vi "Receive.vi"(8 "error in (no error)":errorcluster, 10 "timeout in ms (-1)":i32=-1, 11 "result_from_call in":refnum<class "result_from_call.lvclass">) -> (0 "error out":errorcluster, 2 "timeout":bool, 3 "result_from_call out":refnum<class "result_from_call.lvclass">)   [LabVIEW 2015, in "result_from_call.lvclass"]
uses:
  result_from_call.lvclass
  result_from_call.lvclass/result_from_call.ctl
  result.lvclass
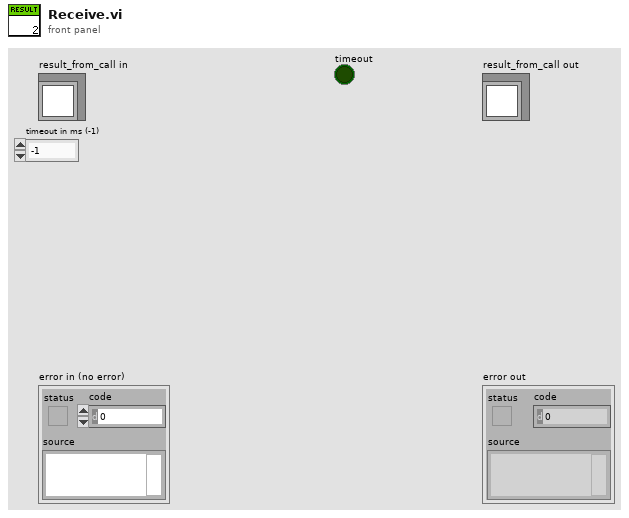
[diagram p1: front panel]
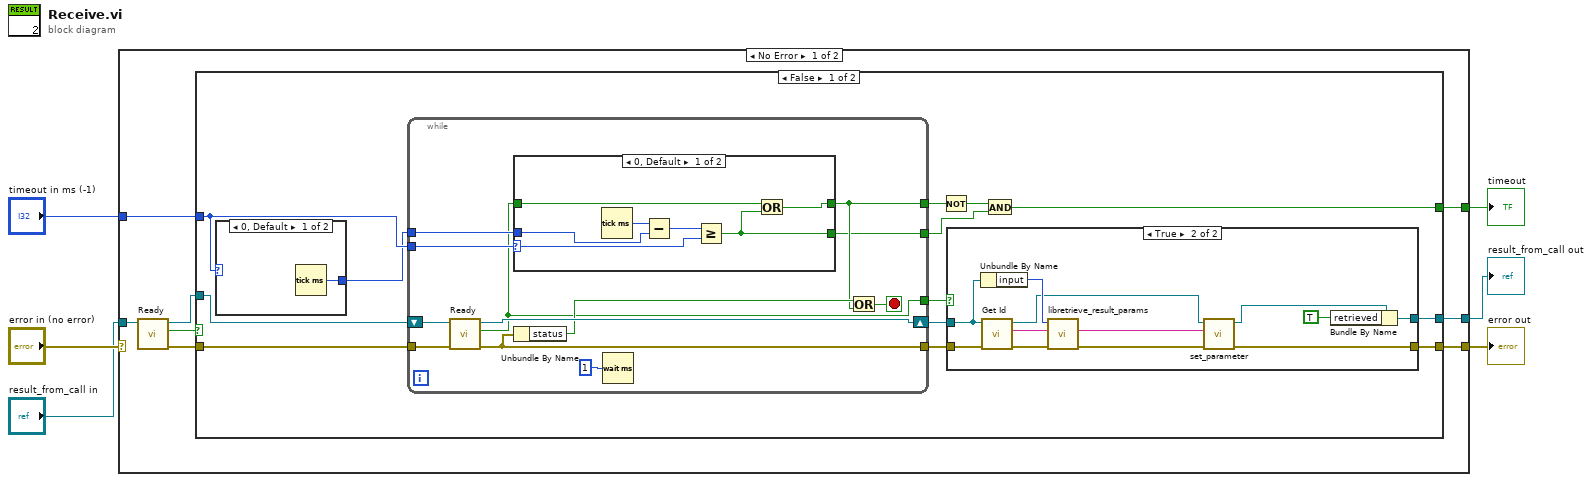
[diagram p0: block diagram]
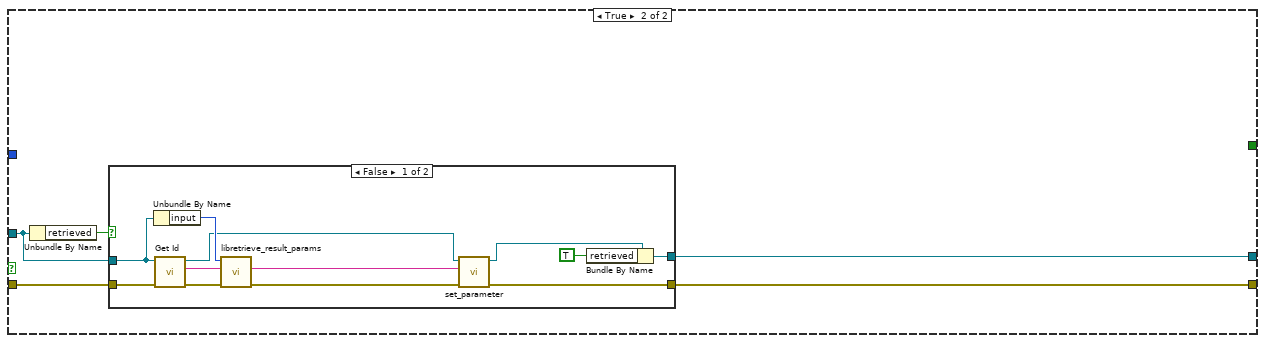
[diagram p5: hidden frame]
diagram:
  n1 = case shown="No Error" "error in (no error)" {
    selector: "error in (no error)" -> [_ w83]
    tunnel: [w13 w83] -> w5
    tunnel: [w12 w82] -> w3
    tunnel: "result_from_call in" -> [w10 w82]
    tunnel: "timeout in ms (-1)" -> [w14 _]
    tunnel: [w11 _] -> w1
    frame No Error {
      n2 = call "Ready.vi"("result_from_call in"=w10) -> ("result_from_call out"=w9:refnum<class "result_from_call.lvclass">, "ready"=w7:bool, "error out"=w8:errorcluster)  [unwired: 7 in]
      n3 = case shown="False" w7 {
        tunnel: w14 -> [w27 _]
        tunnel: [w15 w63] -> w13
        tunnel: [w16 w64] -> w12
        tunnel: [w22 _] -> w11
        tunnel: w9 -> [w21 w65]
        tunnel: w8 -> [w20 w66]
        frame False {
          n4 = case shown="0, Default" w27 {
            tunnel: [w42 _] -> w26
            frame 0, Default {
              n5 = Tick Count (ms)() -> (millisecond timer value=w42:u32)
            }
            frame -1 {
            }
          }
          n6 = while {
            shift-right: [w50] -> w18
            shift-left: w21 -> [w51]
            tunnel: w27 -> [w53]
            tunnel: w26 -> [w52]
            tunnel: [w47] -> w17
            tunnel: [w46] -> w25
            tunnel: [w45] -> w24
            tunnel: w20 -> [w44]
            tunnel: [w43] -> w19
            stop <- w48 stop-if-true
            n7 = call "Ready.vi"("result_from_call in"=w51, "error in (no error)"=w44) -> ("result_from_call out"=w50:refnum<class "result_from_call.lvclass">, "ready"=w43:bool, "error out"=w47:errorcluster)  [unwired: 6 in]
            n8 = case shown="0, Default" w53 {
              selector: w53 -> [w58 _]
              tunnel: w52 -> [w61 _]
              tunnel: w43 -> [w57 w62]
              tunnel: [w56 w62] -> w46
              tunnel: [w55 _] -> w45
              frame 0, Default {
                n9 = Tick Count (ms)() -> (millisecond timer value=w60:u32)
                n10 = Subtract(x=w60, y=w61) -> (x-y=w59:u32)
                n11 = Greater Or Equal?(x=w59, y=w58) -> (x >= y?=w55:bool)
                n12 = Or(x=w57, y=w55) -> (x .or. y?=w56:bool)
              }
              frame -1 {
              }
            }
            n13 = Unbundle By Name(w47) -> ("status"=w49:bool)
            n14 = Wait (ms)(milliseconds to wait=u32 1) -> ()  [unwired: 1 out]
            n15 = Or(x=w49, y=w46) -> (x .or. y?=w48:bool)
          }
          n16 = Not(x=w25) -> (.not. x?=w23:bool)
          n17 = case shown="True" w19 {
            tunnel: w18 -> [w29 w34]
            tunnel: w17 -> [w28 w33]
            tunnel: [w29 w37] -> w16
            tunnel: [w28 w39] -> w15
            frame False {
            }
            frame True {
              n18 = Unbundle By Name(w34) -> ("input"=w35:i32)
              n19 = call "Get Id.vi"("error in (no error)"=w33, "result in"=w34) -> ("error out"=w32:errorcluster, "id"=w31:string, "result out"=w30:refnum<class "result_from_call.lvclass">)  [unwired: 7 in]
              n20 = call "libretrieve_result_params.vi"("error in (no error)"=w32, "id"=w31, "input"=w35) -> ("error out"=w40:errorcluster, "params"=w41:string)  [unwired: 7 in]
              n21 = call "set_parameter.vi"("error in (no error)"=w40, "parameter"=w41, "result in"=w30) -> ("error out"=w39:errorcluster, "result out"=w38:refnum<class "result_from_call.lvclass">)  [unwired: 7 in]
              n22 = Bundle By Name(cluster=w38, "retrieved"=TRUE) -> (w37:refnum<class "result_from_call.lvclass">)
            }
          }
          n23 = And(x=w23, y=w24) -> (x .and. y?=w22:bool)
        }
        frame True {
          n24 = Unbundle By Name(w65) -> ("retrieved"=w67:bool)
          n25 = case shown="False" w67 {
            tunnel: w65 -> [w72 w81]
            tunnel: w66 -> [w71 w80]
            tunnel: [w75 w81] -> w64
            tunnel: [w77 w80] -> w63
            frame False {
              n26 = Unbundle By Name(w72) -> ("input"=w73:i32)
              n27 = call "Get Id.vi"("error in (no error)"=w71, "result in"=w72) -> ("error out"=w70:errorcluster, "id"=w68:string, "result out"=w69:refnum<class "result_from_call.lvclass">)  [unwired: 7 in]
              n28 = call "libretrieve_result_params.vi"("error in (no error)"=w70, "id"=w68, "input"=w73) -> ("error out"=w78:errorcluster, "params"=w79:string)  [unwired: 7 in]
              n29 = call "set_parameter.vi"("error in (no error)"=w78, "parameter"=w79, "result in"=w69) -> ("error out"=w77:errorcluster, "result out"=w76:refnum<class "result_from_call.lvclass">)  [unwired: 7 in]
              n30 = Bundle By Name(cluster=w76, "retrieved"=TRUE) -> (w75:refnum<class "result_from_call.lvclass">)
            }
            frame True {
            }
          }
        }
      }
    }
    frame Error {
    }
  }
  "error out" <- w5
  "result_from_call out" <- w3
  "timeout" <- w1
